vi "AprilTag Target Package Code 3.vi"() -> ()   [LabVIEW 2023]
uses:
  <vilib>/vision/Image Controls.llb/IMAQ Image.ctl
  <vilib>/Utility/config.llb/NI_LVConfig.lvlib
  Camera Set Up/Event/Event Setup Types.ctl
  State Machine/AprialTag States.ctl
  State Machine/AprialTag Main Cluster.ctl
  Steam Type.ctl
  <vilib>/vision/NI_Vision_Development_Module.lvlib
  <vilib>/Utility/config.llb/Write Key (String).vi
  <vilib>/Utility/config.llb/Read Key (String).vi
  <vilib>/ptbypt/NI_PtbyPt.lvlib
  Camera Info.ctl
  <vilib>/vision/Pattern Matching.llb/IMAQ Match Range Setting.ctl
  <vilib>/vision/Shape Detection.llb/ShapeDetectionMatchOptions.ctl
panel:
  in  "Main":enum32{"Page 1", "Page 2"}(tab)
  out "Target Pitch":dbl[](array[numeric]) caption="Tag Pitch (deg)" format="%.1f"
  out "Target Yaw":dbl[](array[numeric]) caption="Tag Yaw (deg)" format="%.1f"
  out "Tag ID":dbl[](array[numeric]) caption="Tag Number"
  out "Image":T1(plugin-control)
  in  "Camera Name":string="cam0"
  in  "Settings":bool
  in  "Save":bool
  in  "Tools":bool
  out "AprilTag Fps":dbl format="%#.0f"
  out "Distance":dbl[](array[numeric]) caption="Tag Distance (in)" format="%.1f"
  out "Angle":dbl[](array[numeric]) caption="Center Angle (deg)" format="%.1f"
  in  "Minimum match score":dbl=100.0
  in  "Home":bool
  in  "Robot Calibration Cluster":T2={"Camera Height on robot (in)"=9.5, "Camera Angle on the robot (deg)"=2.5, "Camera FOV Top to Bottom View Angle (deg)"=26.5, "Camera FOV Left to Right View Angle (deg)"=68.5, "Target size (in)"=6.5, "Distance to front of bumper (in)"=9.75, "Focal Length (mm)"=10.0, "Yaw Slope"=12.276, "Yaw Offset"=2.0} {"Yaw Offset" format="%#_13g"; "Yaw Slope" format="%#_13g"; "Camera FOV Left to Right View Angle (deg)" format="%#_13g"; "Focal Length (mm)" format="%#_13g"; "Distance to front of bumper (in)" format="%#_13g"; "Target size (in)" format="%#_13g"; "Camera FOV Top to Bottom View Angle (deg)" format="%#_13g"; "Camera Angle on the robot (deg)" format="%#_13g"; "Camera Height on robot (in)" format="%#_13g"}
  in  "Max Rect Size (pix)":dbl=1200.0
  in  "Min Rect Size (pix)":dbl=50.0
  in  "Match Options":T3={"Rotation"=TRUE, "Scale"=TRUE, "Occlusion"=FALSE, "Range Settings"=[{"Match Constraints"=0, "Min"=-25.0, "Max"=25.0}, {"Match Constraints"=1, "Min"=25.0, "Max"=200.0}]} {"Range Settings"."Match Constraints" items=["Rotation Angle (degrees)", "Scale Factor (%)", "Occlusion (%)"]}
  # "Edit the camera name to the camera that you are going to use for this target package"
  # "Range"
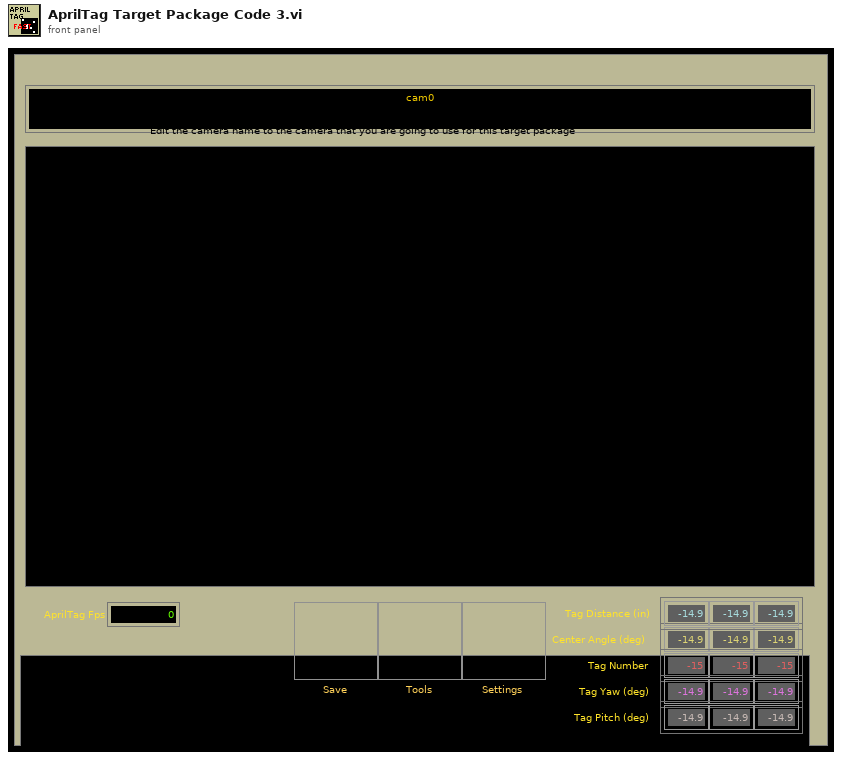
[diagram p1: front panel]
types:
  T1 = typedef "IMAQ Image.ctl" = refnum<image>
  T2 = typedef "Camera Info.ctl" = cluster{"Camera Height on robot (in)":dbl, "Camera Angle on the robot (deg)":dbl, "Camera FOV Top to Bottom View Angle (deg)":dbl, "Camera FOV Left to Right View Angle (deg)":dbl, "Target size (in)":dbl, "Distance to front of bumper (in)":dbl, "Focal Length (mm)":dbl, "Yaw Slope":dbl, "Yaw Offset":dbl}
  T3 = typedef "ShapeDetectionMatchOptions.ctl" = cluster{"Rotation":bool, "Scale":bool, "Occlusion":bool, "Range Settings":T4[]}
  T4 = typedef "IMAQ Match Range Setting.ctl" = cluster{"Match Constraints":u32, "Min":dbl, "Max":dbl}
  T5 = typedef "AprialTag States.ctl" = enum16{"Message Dispatcher", "INI", "Open", "Save", "Exit"}
  T6 = typedef "AprialTag Main Cluster.ctl" = cluster{"AprilTage FIFO":T5[], "Camera Name":string, "AprilTag path":path, "Control Ref's":refnum<vi>[], "Main Image":T1, "Intensity Mask":T1, "Resize Mask":T1, "Timeout":i32, "EDIT Settings":bool, "Calibration path":path, "Camera Number":dbl}
  T7 = cluster{"Min Width":dbl, "Max Width":dbl, "Min Height":dbl, "Max Height":dbl}
  T8 = typedef "Steam Type.ctl" = enum8{"Unknown", "Apriltag", "Algae", "Coral"}
  T9 = typedef "Event Setup Types.ctl" = enum16{"Default", "Camera Loop Started", "Close Settings", "GreyScale", "Open Front Panel", "Reset Team Number", "Save Data", "Exit"}
  T10 = cluster{"Corners":cluster{"X":sgl, "Y":sgl}[], "Angle":dbl, "Width":dbl, "Height":dbl, "Score":dbl}[]
  T11 = typedef "AprilTag Target Fields.ctl" = cluster{"diameter points":cluster{"first point":cluster{"x":dbl, "y":dbl}, "projected point":cluster{"x":dbl, "y":dbl}}, "normalized center":cluster{"x":dbl, "y":dbl}, "Overall Score":dbl, "Distance (ft)":dbl, "Offset Angle":dbl, "Tag corner points":cluster{"X":dbl, "Y":dbl}[], "Tag Center":cluster{"X":dbl, "Y":dbl}, "Tag Yaw":dbl, "Tag Pitch":dbl, "Target Roll (deg)":dbl, "AprilTag Number":i32, "homography matrix":dbl[]}
  T12 = typedef "Image Type" = u32
  T13 = typedef "NI_LVConfig.lvlib/Config Data RefNum.ctl" = refnum<k1>
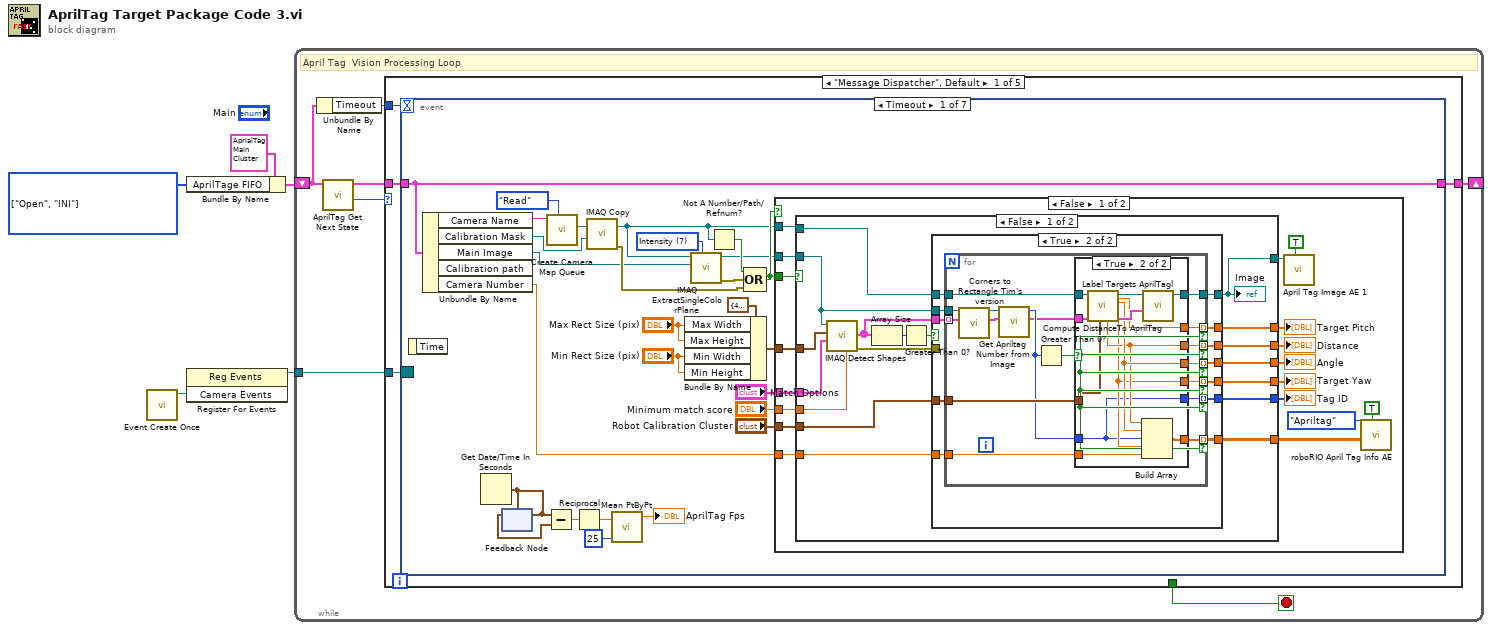
[diagram p0: block diagram]
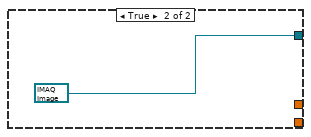
[diagram p4: hidden frame]
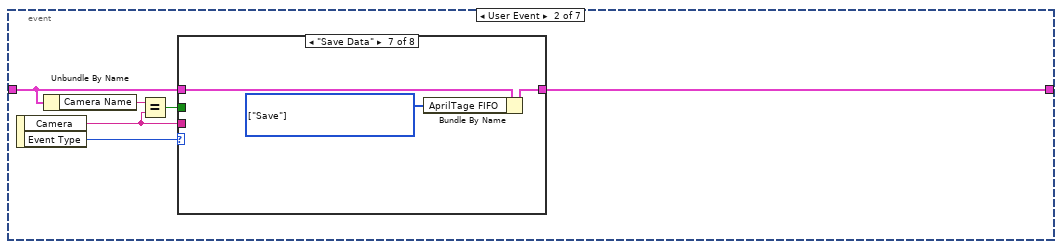
[diagram p6: hidden frame]
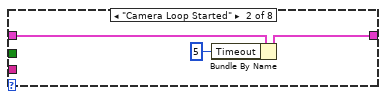
[diagram p8: hidden frame]
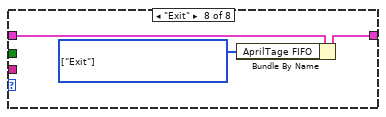
[diagram p13: hidden frame]
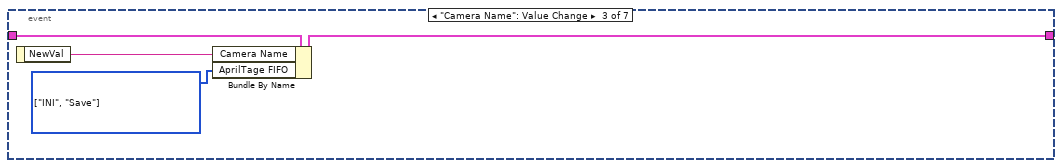
[diagram p14: hidden frame]
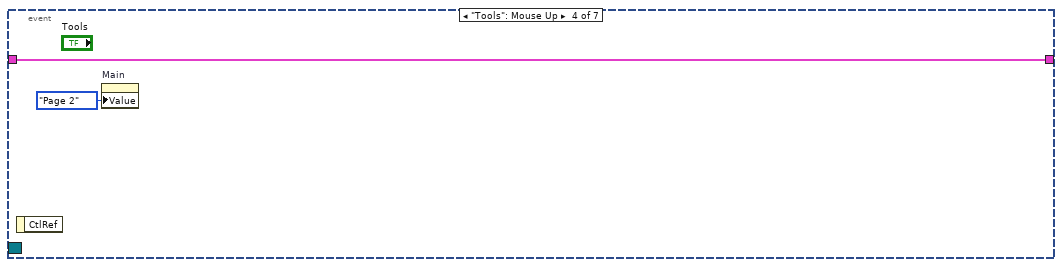
[diagram p15: hidden frame]
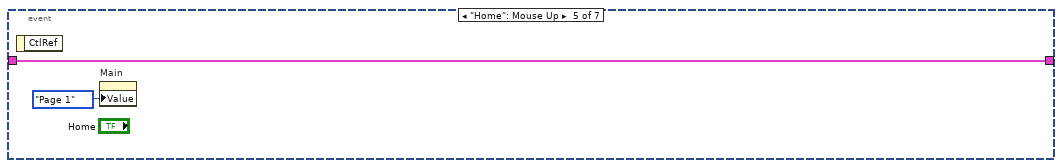
[diagram p16: hidden frame]
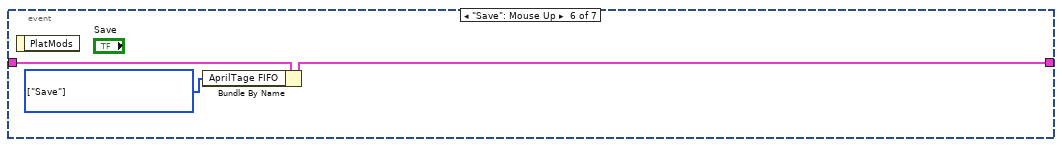
[diagram p17: hidden frame]
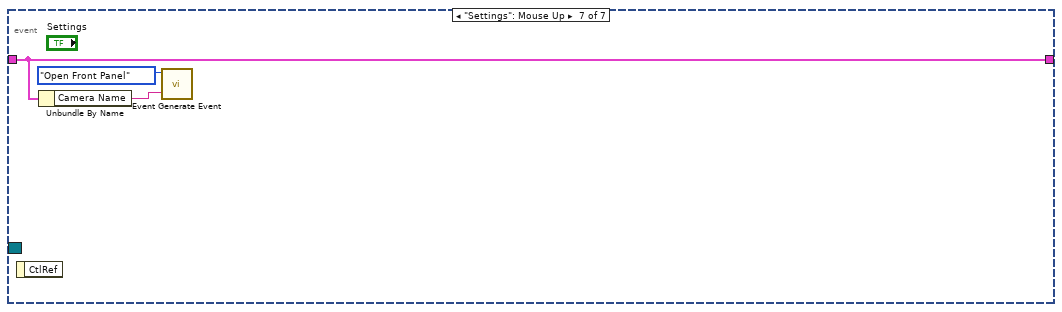
[diagram p18: hidden frame]
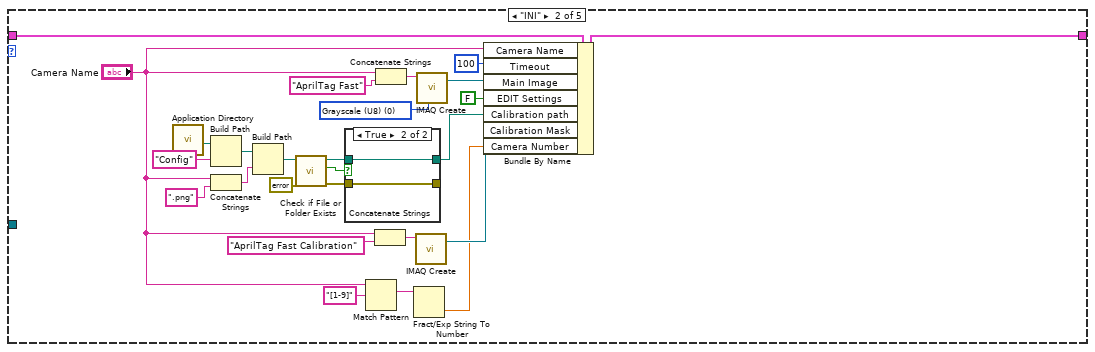
[diagram p19: hidden frame]
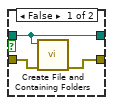
[diagram p20: hidden frame]
diagram:
  w1 = T5[] [enum."Open", enum."INI"] items=["Message Dispatcher", "INI", "Open", "Save", "Exit"] ("AprilTage FIFO")
  n1 = call "Event Create Once.vi"() -> ("Camera Events"=w5:refnum<user-event>)  [unwired: 10 in, 1 out]
  n2 = Bundle By Name(cluster=T6 {"AprilTage FIFO"=[], "Camera Name"="", "AprilTag path"=path "", "Control Ref's"=[], "Main Image"=refnum, "Intensity Mask"=refnum, "Resize Mask"=refnum, "Timeout"=5, "EDIT Settings"=FALSE, "Calibration path"=path "", "Camera Number"=0.0} ("AprilTag Main Cluster out"), "AprilTage FIFO"=w1) -> (w2:T6)
  n3 = register-events(w5) -> (reference out=w4:refnum<event-registration>)  [unwired: 2 in, 1 out]
  n4 = while {
    tunnel: w4 -> [w12]
    shift-right: [w8] -> _
    shift-left: w2 -> [w6]
    stop <- w11 stop-if-true
    # "April Tag  Vision Processing Loop"
    n5 = Unbundle By Name(w6) -> ("Timeout"=w7:i32)
    n6 = call "AprilTag Get Next State.vi"("AprilTag Main Cluster in"=w6) -> ("Next State"=w9:T5, "AprilTag Main Cluster out"=w10:T6)  [unwired: 9 in]
    n7 = case shown="\"Message Dispatcher\", Default" w9 {
      tunnel: w12 -> [w16 _ _ _ _]
      tunnel: [_ _ _ _ TRUE] -> w11
      tunnel: w10 -> [w14 w183 w204 w242 w259]
      tunnel: [w15 w182 w202 w242 w259] -> w8
      tunnel: w7 -> [w13 _ _ _ _]
      frame "Message Dispatcher", Default {
        n8 = event shown="[0] Timeout" {
          selector: w16 -> [_ _ _ _ _ _ _]
          dyn-events: _ -> [_ _ _ _ _ _ _]
          timeout: w13 -> [_ _ _ _ _ _ _]
          tunnel: w14 -> [w43 w127 w147 w148 w150 w154 w156]
          tunnel: [w43 w129 w146 w148 w150 w153 w156] -> w15
          event Timeout {
            w20 = 7 items=["Red", "Green", "Blue", "Hue", "Saturation", "Luminance", "Value", "Intensity"] ("Color Plane")
            n9 = event-data() -> ()  [unwired: 1 in, 1 out]
            n10 = Unbundle By Name(w43) -> ("Camera Name"=w41:string, "Calibration Mask"=w23:T1, "Main Image"=w19:T1, "Camera Number"=w40:dbl)  [unwired: 1 out]
            n11 = Get Date/Time In Seconds() -> (seconds since 1Jan1904=w29:timestamp)
            n12 = feedback-in #1(w29) -> ()
            n13 = feedback #1(w29) -> (w30:timestamp)
            n14 = Subtract(x=w29, y=w30) -> (x-y=w28:dbl)
            n15 = call "Create Camera Map Queue.vi"("Action"=enum16{"Read", "Write"}."Read", "Camera"=w41) -> ("Image out"=w24:T1)  [unwired: 8 in, 1 out]
            n16 = Reciprocal(x=w28) -> (1/x=w27:dbl)
            n17 = call "IMAQ Copy"("Image Dst"=w23, "Image Src"=w24) -> ("error out"=w22:errorcluster, "Image Dst Out"=w21:T1)  [unwired: 4 in]
            n18 = call <vilib>:"Mean PtByPt.vi"("x"=w27, "sample length"=25) -> ("mean"=→"AprilTag Fps":dbl)  [unwired: 2 in, 1 out]
            n19 = Bundle By Name(cluster=T7 {"Min Width"=40.0, "Max Width"=100.0, "Min Height"=40.0, "Max Height"=200.0} ("Rectangle Descriptor"), "Max Width"="Max Rect Size (pix)", "Max Height"="Max Rect Size (pix)", "Min Width"="Min Rect Size (pix)", "Min Height"="Min Rect Size (pix)") -> (w39:T7)
            n20 = call "IMAQ ExtractSingleColorPlane"("Color Plane"=w20, "Image Dst"=w19, "Image Src"=w21) -> ("error out"=w17:errorcluster, "Image Dst Out"=w18:T1)  [unwired: 7 in]
            n21 = Not A Number/Path/Refnum?(number/path/refnum=w21) -> (NaN/Path/Refnum?=w32:bool)
            n22 = Compound Arithmetic op=OR(w32, w17, w22) -> (w31:bool)
            n23 = case shown="False" w31 {
              tunnel: "Robot Calibration Cluster" -> [w58 _]
              tunnel: w31 -> [w52 _]
              tunnel: w21 -> [w51 _]
              tunnel: w40 -> [w50 _]
              tunnel: w39 -> [w48 _]
              tunnel: "Match Options" -> [w47 _]
              tunnel: w18 -> [w46 _]
              tunnel: "Minimum match score" -> [w45 _]
              frame False {
                n24 = case shown="False" w52 {
                  tunnel: w58 -> [w79 _]
                  tunnel: [w77 _] -> w60
                  tunnel: [w76 _] -> w57
                  tunnel: [w75 _] -> w56
                  tunnel: [w74 _] -> w55
                  tunnel: [w73 _] -> w54
                  tunnel: [w72 _] -> w53
                  tunnel: w51 -> [w62 _]
                  tunnel: w50 -> [w71 _]
                  tunnel: [w70 T1 refnum ("Image out")] -> w49
                  tunnel: w48 -> [w69 _]
                  tunnel: w47 -> [w66 _]
                  tunnel: w46 -> [w63 _]
                  tunnel: w45 -> [w65 _]
                  frame False {
                    n25 = call-poly "IMAQ Detect Shapes"("Minimum match score"=w65, "Match Options"=w66, "Rectangle Descriptor"=w69, "Image"=w63) -> ("error out"=w67:errorcluster, "Rectangles"=w68:T10)  [unwired: 5 in, 1 out]
                    n26 = Array Size(array=w68) -> (size(s)=w64:i32)
                    n27 = Greater Than 0?(x=w64) -> (x > 0?=w78:bool)
                    n28 = case shown="True" w78 {
                      tunnel: w62 -> [w80 w81]
                      tunnel: w68 -> [_ w92]
                      tunnel: [w80 w83] -> w70
                      tunnel: w79 -> [_ w91]
                      tunnel: [_ w90] -> w77
                      tunnel: [_ w89] -> w76
                      tunnel: [_ w88] -> w75
                      tunnel: [_ w87] -> w74
                      tunnel: [_ w86] -> w73
                      tunnel: [_ w85] -> w72
                      tunnel: w71 -> [_ w84]
                      tunnel: w67 -> [_ _]
                      tunnel: w63 -> [_ w82]
                      frame False {
                      }
                      frame True {
                        n29 = for {
                          tunnel: w92 -> [w107] mode=indexing
                          tunnel: w81 -> [w99]
                          tunnel: [w108] -> w83
                          tunnel: [w93] -> w87 mode=indexing if=w94
                          tunnel: [w104] -> w85 mode=indexing if=w94
                          tunnel: [w106] -> w86 mode=indexing if=w94
                          tunnel: w91 -> [w105]
                          tunnel: [w103] -> w88 mode=indexing if=w94
                          tunnel: [w102] -> w90 mode=indexing if=w94
                          tunnel: [w101] -> w89 mode=indexing if=w94
                          tunnel: w84 -> [w100]
                          tunnel: w82 -> [w97]
                          n30 = call "Corners to Rectangle Tim's version.vi"("Rectangle Descriptor"=w107) -> ("tag info out"=w96:T11)  [unwired: 10 in]
                          n31 = call "Get Apriltag Number from Image.vi"("tag info"=w96, "Image"=w97) -> ("tag info out"=w95:T11, "AprilTag#"=w98:i32)  [unwired: 7 in, 1 out]
                          n32 = Greater Than 0?(x=w98) -> (x > 0?=w94:bool)
                          n33 = case shown="True" w94 {
                            tunnel: [w109 w122] -> w108
                            tunnel: w95 -> [_ w121]
                            tunnel: [_ w118] -> w106
                            tunnel: w105 -> [_ w117]
                            tunnel: [_ w116] -> w104
                            tunnel: [_ w115] -> w103
                            tunnel: [_ w114] -> w102
                            tunnel: [_ w113] -> w101
                            tunnel: w100 -> [_ w112]
                            tunnel: w99 -> [w109 w111]
                            tunnel: w98 -> [_ w110]
                            tunnel: [_ w110] -> w93
                            frame False {
                            }
                            frame True {
                              n34 = call "Compute DistanceTo AprilTag.vi"("Robot Calibration Cluster"=w117, "results"=w121, "Image Src"=w111) -> ("results out"=w120:T11, "Target Yaw (deg)"=w115:dbl, "Offset Angle"=w118:dbl, "Image Dst Out"=w119:T1, "Distance from target (in)"=w116:dbl, "Target Pitch (deg)"=w113:dbl)  [unwired: 2 in, 1 out]
                              n35 = Build Array(w116, w118, w110, w115, w112) -> (w114:dbl[])
                              n36 = call "Label Targets AprilTagl.vi"("results"=w120, "Image in"=w119) -> ("Image out"=w122:T1)  [unwired: 9 in]
                            }
                          }
                        }
                      }
                    }
                    "Image" <- w70
                  }
                  frame True {
                  }
                }
                "Distance" <- w53
                "Angle" <- w54
                "Tag ID" <- w55
                "Target Yaw" <- w56
                "Target Pitch" <- w57
                n37 = call "April Tag Image AE 1.vi"("Update"=TRUE, "Ball Image in"=w49) -> ()  [unwired: 9 in, 1 out]
                n38 = call "roboRIO April Tag Info AE.vi"("Update"=TRUE, "Info in"=w60, "Stream Type"=Steam_Type."Apriltag") -> ()  [unwired: 8 in, 1 out]
              }
              frame True {
              }
            }
          }
          event User Event {
            n39 = event-data() -> ("Camera"=w124:string, "Event Type"=w128:T9)  [unwired: 1 in]
            n40 = Unbundle By Name(w127) -> ("Camera Name"=w126:string)
            n41 = Equal?(x=w126, y=w124) -> (x = y?=w125:bool)
            n42 = case shown="\"Save Data\"" w128 {
              tunnel: w127 -> [w130 w133 w134 w135 w136 w137 w140 w143]
              tunnel: [w130 w132 w134 w135 w136 w137 w139 w142] -> w129
              tunnel: w125 -> [_ _ _ _ _ _ _ _]
              tunnel: w124 -> [_ _ _ _ _ _ _ _]
              frame "Default" {
              }
              frame "Camera Loop Started" {
                n43 = Bundle By Name(cluster=w133, "Timeout"=5) -> (w132:T6)
              }
              frame "Close Settings" {
              }
              frame "GreyScale" {
              }
              frame "Open Front Panel" {
              }
              frame "Reset Team Number" {
              }
              frame "Save Data" {
                w138 = T5[] [enum."Save"] items=["Message Dispatcher", "INI", "Open", "Save", "Exit"] ("AprilTage FIFO")
                n44 = Bundle By Name(cluster=w140, "AprilTage FIFO"=w138) -> (w139:T6)
              }
              frame "Exit" {
                w141 = T5[] [enum."Exit"] items=["Message Dispatcher", "INI", "Open", "Save", "Exit"] ("AprilTage FIFO")
                n45 = Bundle By Name(cluster=w143, "AprilTage FIFO"=w141) -> (w142:T6)
              }
            }
          }
          event "Camera Name": Value Change {
            w145 = T5[] [enum."INI", enum."Save"] items=["Message Dispatcher", "INI", "Open", "Save", "Exit"] ("AprilTage FIFO")
            n46 = event-data() -> ("NewVal"=w144:string)  [unwired: 1 in]
            n47 = Bundle By Name(cluster=w147, "Camera Name"=w144, "AprilTage FIFO"=w145) -> (w146:T6)
          }
          event "Tools": Mouse Up {
            n48 = event-data() -> ()  [unwired: 1 in, 1 out]
            n49 = property on="Main" class="TabCtl (strict)"("Value"=enum32{"Page 1", "Page 2"}."Page 2" ("Main")) -> ()  [unwired: 2 in, 2 out]
          }
          event "Home": Mouse Up {
            n50 = event-data() -> ()  [unwired: 1 in, 1 out]
            n51 = property on="Main" class="TabCtl (strict)"("Value"=enum32{"Page 1", "Page 2"}."Page 1" ("Main")) -> ()  [unwired: 2 in, 2 out]
          }
          event "Save": Mouse Up {
            w152 = T5[] [enum."Save"] items=["Message Dispatcher", "INI", "Open", "Save", "Exit"] ("AprilTage FIFO")
            n52 = event-data() -> ()  [unwired: 1 in, 1 out]
            n53 = Bundle By Name(cluster=w154, "AprilTage FIFO"=w152) -> (w153:T6)
          }
          event "Settings": Mouse Up {
            n54 = event-data() -> ()  [unwired: 1 in, 1 out]
            n55 = Unbundle By Name(w156) -> ("Camera Name"=w155:string)
            n56 = call "Event Generate Event.vi"("Camera Name"=w155, "Event Type"=Event_Setup_Types."Open Front Panel") -> ()  [unwired: 10 in]
          }
        }
      }
      frame "INI" {
        w180 = T12 0 items=["Grayscale (U8)", "Grayscale (I16)", "Grayscale (SGL)", "Complex (CSG)", "RGB (U32)", "HSL (U32)", "RGB (U64)", "Grayscale (U16)"] ("Image Type")
        n57 = call <vilib>:"Application Directory.vi"() -> ("Application Directory"=w173:path)
        n58 = Build Path(base path=w173, name or relative path="Config") -> (appended path=w171:path)
        n59 = Concatenate Strings("Camera Name", ".png" ("name or relative path")) -> (w175:string)
        n60 = Build Path(base path=w171, name or relative path=w175) -> (appended path=w170:path)
        n61 = call <vilib>:"Check if File or Folder Exists.vi"("error in (no error)"=errorcluster {"status"=FALSE, "code"=0, "source"=""}, "path"=w170) -> ("error out"=w167:errorcluster, "file or folder exists?"=w168:bool, "dup path"=w169:path)  [unwired: 7 in]
        n62 = case shown="True" w168 {
          tunnel: [w186 w187] -> _
          tunnel: w169 -> [w185 w188]
          tunnel: [w185 w188] -> w165
          tunnel: w167 -> [w184 w187]
          frame False {
            n63 = call <vilib>:"Create File and Containing Folders.vi"("error in (no error)"=w184, "file path"=w185) -> ("error out"=w186:errorcluster)  [unwired: 8 in, 1 out]
          }
          frame True {
          }
        }
        n64 = Match Pattern(string="Camera Name", regular expression="[1-9]") -> (match substring=w160:string)  [unwired: 1 in, 3 out]
        n65 = Concatenate Strings("Camera Name", "AprilTag Fast Calibration" ("string")) -> (w163:string)
        n66 = Concatenate Strings("Camera Name", "AprilTag Fast" ("string")) -> (w179:string)
        n67 = Fract/Exp String To Number(string=w160) -> (number=w159:dbl)  [unwired: 3 in, 1 out]
        n68 = call "IMAQ Create"("Image Name"=w163) -> ("New Image"=w162:T1)  [unwired: 3 in, 2 out]
        n69 = call "IMAQ Create"("Image Name"=w179, "Image Type"=w180) -> ("New Image"=w177:T1)  [unwired: 2 in, 2 out]
        n70 = Bundle By Name(cluster=w183, "Camera Name"="Camera Name", "Timeout"=100, "Main Image"=w177, "EDIT Settings"=FALSE, "Calibration path"=w165, "Calibration Mask"=w162, "Camera Number"=w159) -> (w182:T6)
      }
      frame "Open" {
        n71 = call <vilib>:"Application Directory.vi"() -> ("Application Directory"=w207:path)
        n72 = Build Path(base path=w207, name or relative path="Config") -> (appended path=w205:path)
        n73 = Concatenate Strings("Airtag1" ("string"), ".ini" ("name or relative path")) -> (w217:string)
        n74 = Build Path(base path=w205, name or relative path=w217) -> (appended path=w198:path)
        n75 = call <vilib>:"Check if File or Folder Exists.vi"("error in (no error)"=errorcluster {"status"=FALSE, "code"=0, "source"=""}, "path"=w198) -> ("error out"=w194:errorcluster, "file or folder exists?"=w196:bool, "dup path"=w197:path)  [unwired: 7 in]
        n76 = control-ref of="Main"() -> (w212:refnum<vi>)
        n77 = case shown="False" w196 {
          tunnel: [w220 w221] -> w208
          tunnel: w197 -> [w219 w222]
          tunnel: [w219 w222] -> w195
          tunnel: w194 -> [w218 w221]
          frame False {
            n78 = call <vilib>:"Create File and Containing Folders.vi"("error in (no error)"=w218, "file path"=w219) -> ("error out"=w220:errorcluster)  [unwired: 8 in, 1 out]
          }
          frame True {
          }
        }
        n79 = control-ref of="Robot Calibration Cluster"() -> (w211:refnum<vi>)
        n80 = control-ref of="Match Options"() -> (w192:refnum<vi>)
        n81 = control-ref of="Minimum match score"() -> (w191:refnum<vi>)
        n82 = control-ref of="Max Rect Size (pix)"() -> (w190:refnum<vi>)
        n83 = control-ref of="Min Rect Size (pix)"() -> (w189:refnum<vi>)
        n84 = control-ref of="Camera Name"() -> (w203:refnum<vi>)
        n85 = Build Array(w212, w211, w203, w192, w191, w190, w189) -> (w201:refnum<vi>[])
        n86 = call <vilib>:"Open Config Data.vi"("error in (no error)"=w208, "configuration file path"=w195) -> ("error out"=w213:errorcluster, "refnum"=w216:T13)  [unwired: 7 in, 1 out]
        n87 = for {
          tunnel: "Info" ("Camera Name") -> [w235]
          tunnel: w201 -> [w233] mode=indexing
          shift-right: [w237] -> w215
          shift-left: w216 -> [w238]
          shift-right: [w236] -> w214
          shift-left: w213 -> [w234]
          tunnel: [w228] -> _ mode=indexing
          tunnel: errorcluster {"status"=FALSE, "code"=0, "source"=""} ("error out") -> [w227]
          tunnel: [w223] -> _ mode=indexing
          n88 = property class="Ctl"(reference=w233, error in=w227) -> (reference out=w231:refnum<vi>, error out=w229:errorcluster, "Label.Text"=w232:string, "Value"=w225:variant)
          n89 = Variant To Flattened String(Variant=w225) -> (1:w224:i16[])  [unwired: 1 out]
          n90 = call-poly <vilib>:"Read Key.vi"("section"=w235, "error in (no error)"=w234, "key"=w232, "refnum"=w238) -> ("error out"=w236:errorcluster, "value"=w230:string, "refnum out"=w237:T13)  [unwired: 4 in, 1 out]
          n91 = Flattened String To Variant(6:w230, 7:w224) -> (0:w223:errorcluster, 3:w226:variant)  [unwired: 1 in]
          n92 = property class="Ctl"(reference=w231, error in=w229, "Value"=w226) -> (error out=w228:errorcluster)  [unwired: 1 out]
        }
        n93 = call <vilib>:"Close Config Data.vi"("error in (no error)"=w214, "refnum"=w215) -> ()  [unwired: 8 in, 2 out]
        n94 = Bundle By Name(cluster=w204, "Control Ref's"=w201, "AprilTag path"=w195) -> (w202:T6)
      }
      frame "Save" {
        n95 = Unbundle By Name(w242) -> ("Control Ref's"=w240:refnum<vi>[], "AprilTag path"=w241:path)
        n96 = call <vilib>:"Open Config Data.vi"("configuration file path"=w241) -> ("error out"=w243:errorcluster, "refnum"=w246:T13)  [unwired: 8 in, 1 out]
        n97 = for {
          tunnel: "Info" ("Camera Name") -> [w252]
          shift-right: [w255] -> w245
          shift-left: w246 -> [w256]
          shift-right: [w254] -> w244
          shift-left: w243 -> [w253]
          tunnel: w240 -> [w247] mode=indexing
          n98 = property class="Ctl"(reference=w247, error in=w253) -> (error out=w249:errorcluster, "Label.Text"=w251:string, "Value"=w250:variant)  [unwired: 1 out]
          n99 = Variant To Flattened String(Variant=w250) -> (data string=w248:string)  [unwired: 1 out]
          n100 = call-poly <vilib>:"Write Key.vi"("section"=w252, "error in (no error)"=w249, "value"=w248, "key"=w251, "refnum"=w256) -> ("error out"=w254:errorcluster, "refnum out"=w255:T13)  [unwired: 4 in, 1 out]
        }
        n101 = call <vilib>:"Close Config Data.vi"("error in (no error)"=w244, "refnum"=w245) -> ()  [unwired: 8 in, 2 out]
      }
      frame "Exit" {
        n102 = Unbundle By Name(w259) -> ("Calibration Mask"=w258:T1, "Main Image"=w257:T1)
        n103 = call "IMAQ Dispose"("Image"=w258) -> ()  [unwired: 5 in, 1 out]
        n104 = call "IMAQ Dispose"("Image"=w257) -> ()  [unwired: 5 in, 1 out]
      }
    }
  }
